vi "Read List Step Parameter.vi"(8 "error in (no error)":errorcluster, 10 "List Step Number(0)":dbl, 11 "VISA resource name":refnum<visa-resource-name>) -> (0 "error out":errorcluster, 1 "Step Timing":string, 2 "Number of Steps":string, 3 "VISA resource name out":refnum<visa-resource-name>)   [LabVIEW 2021, in "Keithley 2200 Series.lvlib"]
doc: "Reads the parameter configured in a list step based on the Step number."
uses:
  <instrlib>/Keithley 2200 Series/Keithley 2200 Series.lvlib
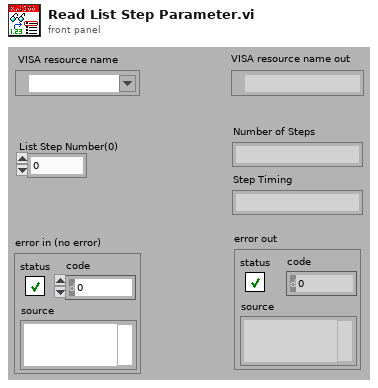
[diagram p1: front panel]
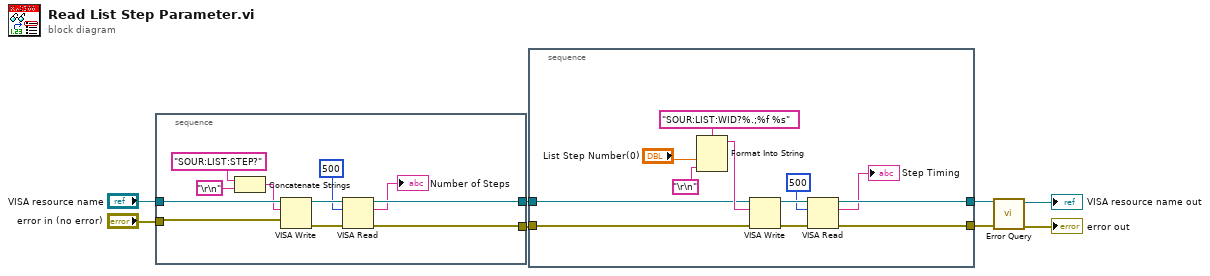
[diagram p0: block diagram]
diagram:
  n1 = stacked-sequence {
    tunnel: [w14] -> w5
    tunnel: "error in (no error)" -> [w19]
    tunnel: [w15] -> w7
    tunnel: "VISA resource name" -> [w10]
    frame #0 {
      n2 = Concatenate Strings("SOUR:LIST:STEP?" ("format string"), "\r\n" ("End of Line Constant")) -> (w9:string)
      n3 = VISA Write(VISA resource name=w10, write buffer=w9, error in (no error)=w19) -> (VISA resource name out=w18:refnum<visa-resource-name>, error out=w17:errorcluster)  [unwired: 1 out]
      n4 = VISA Read(VISA resource name=w18, byte count=u32 500, error in (no error)=w17) -> (VISA resource name out=w15:refnum<visa-resource-name>, read buffer=→"Number of Steps":string, error out=w14:errorcluster)  [unwired: 1 out]
    }
  }
  n5 = stacked-sequence {
    tunnel: w7 -> [w29]
    tunnel: [w24] -> w4
    tunnel: [w23] -> w3
    tunnel: w5 -> [w27]
    frame #0 {
      n6 = Format Into String(format string="SOUR:LIST:WID?%.;%f %s", "List Step Number(0)", "\r\n" ("End of Line Constant")) -> (resulting string=w30:string)  [unwired: 2 in, 1 out]
      n7 = VISA Write(VISA resource name=w29, write buffer=w30, error in (no error)=w27) -> (VISA resource name out=w25:refnum<visa-resource-name>, error out=w26:errorcluster)  [unwired: 1 out]
      n8 = VISA Read(VISA resource name=w25, byte count=u32 500, error in (no error)=w26) -> (VISA resource name out=w24:refnum<visa-resource-name>, read buffer=→"Step Timing":string, error out=w23:errorcluster)  [unwired: 1 out]
    }
  }
  n9 = call <instrlib>:"Error Query.vi"("error in (no error)"=w3, "VISA resource name"=w4) -> ("error out"=→"error out":errorcluster, "VISA resource name out"=→"VISA resource name out":refnum<visa-resource-name>)  [unwired: 8 out]
